vi "Destroy Event.vi"(8 "error in (no error)":errorcluster, 11 "Event in":refnum<class "Event.lvclass">) -> (0 "error out":errorcluster)   [LabVIEW 2009, in "EventManagerLibrary.lvlib" / "Event.lvclass"]
doc: "This vi runs normally even if an error occurred before this vi."
uses:
  Event.lvclass
  Event.lvclass/Event.ctl
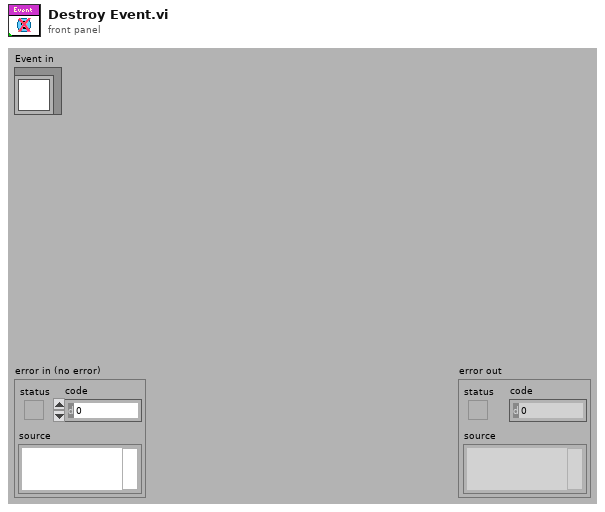
[diagram p1: front panel]
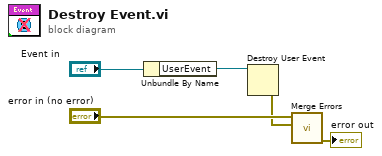
[diagram p0: block diagram]
diagram:
  n1 = Unbundle By Name("Event in") -> ("UserEvent"=w1:refnum<user-event>)
  n2 = Destroy User Event(user event=w1) -> (error out=w2:errorcluster)  [unwired: 1 in]
  n3 = call <vilib>:"Merge Errors.vi"("error in 2 (no error)"=w2, "error in 1 (no error)"="error in (no error)") -> ("error out"=→"error out":errorcluster)  [unwired: 2 in, 3 out]
